vi "Connect - Instrument Only.vi"(8 "error in (no error)":errorcluster, 11 "PXIe5413 in":refnum<class "PXIe5413.lvclass">) -> (0 "error out":errorcluster, 3 "PXIe5413 out":refnum<class "PXIe5413.lvclass">)   [LabVIEW 2018, in "PXIe5413.lvlib" / "PXIe5413.lvclass"]
uses:
  PXIe5413.lvclass
  PXIe5413.lvclass/PXIe5413.ctl
  PPLs/Function Generator/Parent/Function Generator.lvlibp/Function Generator.lvclass
  C:/Projects/LabVIEW/PPLs/Function Generator/Parent/Function Generator.lvlibp/Function Generator.lvclass
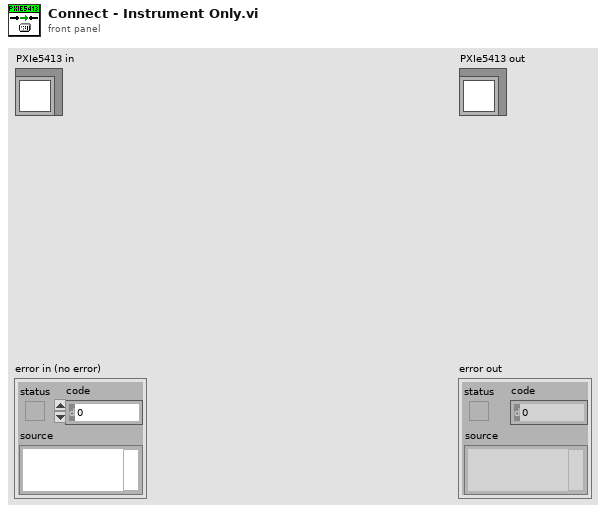
[diagram p1: front panel]
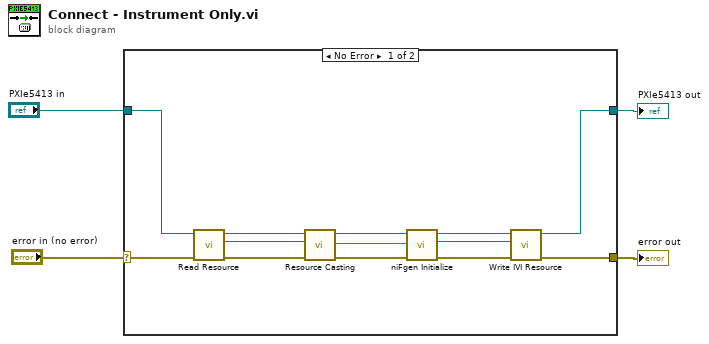
[diagram p0: block diagram]
diagram:
  n1 = case shown="No Error" "error in (no error)" {
    selector: "error in (no error)" -> [w16 w18]
    tunnel: [w5 w18] -> w3
    tunnel: [w6 w17] -> w2
    tunnel: "PXIe5413 in" -> [w15 w17]
    frame No Error {
      n2 = call "Read Resource.vi"("error in (no error)"=w16, "Function Generator in"=w15) -> ("error out"=w14:errorcluster, "Resource"=w7:refnum<visa-resource-name>, "Function Generator out"=w13:refnum<class "PXIe5413.lvclass">)  [unwired: 7 in]
      n3 = call "Resource Casting.vi"("error in (no error)"=w14, "VISA Resource In"=w7, "PXIe5413 in"=w13) -> ("error out"=w11:errorcluster, "Casted Resource"=w12:string, "PXIe5413 out"=w8:refnum<class "PXIe5413.lvclass">)  [unwired: 6 in]
      n4 = call <instrlib>:"niFgen Initialize.vi"("error in (no error)"=w11, "Resource Name"=w12) -> ("error out"=w9:errorcluster, "Instrument Handle Out"=w10:refnum<k15>)  [unwired: 8 in]
      n5 = call "Write IVI Resource.vi"("error in (no error)"=w9, "IVI Resource"=w10, "PXIe5413 in"=w8) -> ("error out"=w5:errorcluster, "PXIe5413 out"=w6:refnum<class "PXIe5413.lvclass">)  [unwired: 7 in]
    }
    frame Error {
    }
  }
  "error out" <- w3
  "PXIe5413 out" <- w2
